vi "Write Best Cost.vi"(8 "error in (no error)":errorcluster, 10 "Best Cost":u64, 11 "State Value in":refnum<class "State Value.lvclass">) -> (0 "error out":errorcluster, 3 "State Value out":refnum<class "State Value.lvclass">)   [LabVIEW 2019, in "23.lvlib" / "State Value.lvclass"]
uses:
  State Value.lvclass
  State Value.lvclass/State Value.ctl
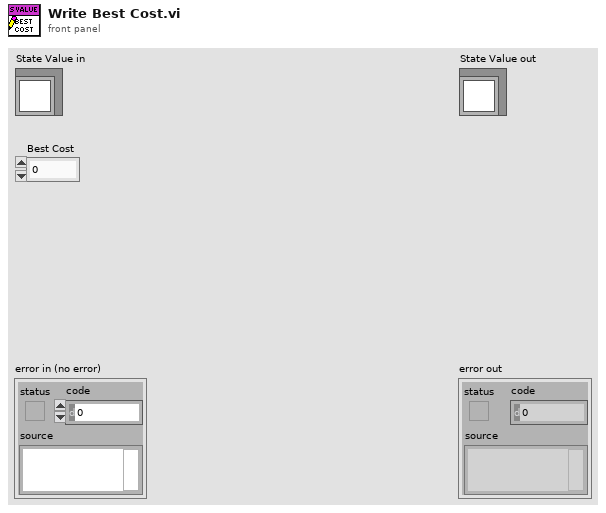
[diagram p1: front panel]
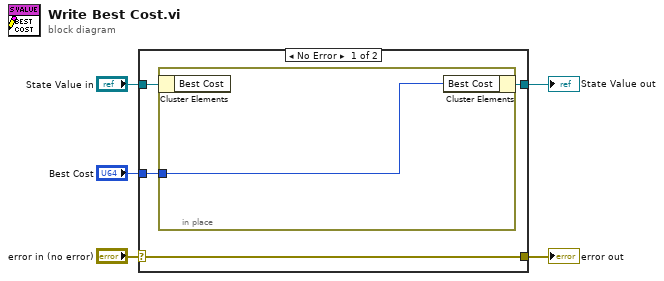
[diagram p0: block diagram]
diagram:
  n1 = case shown="No Error" "error in (no error)" {
    selector: "error in (no error)" -> [w9 w11]
    tunnel: [w9 w11] -> w4
    tunnel: [w7 w12] -> w2
    tunnel: "State Value in" -> [w6 w12]
    tunnel: "Best Cost" -> [w8 _]
    frame No Error {
      n2 = in-place {
        in-place-border: w8 -> [w10]
        n3 = in-place-cluster #1(w6) -> ()  [unwired: 1 out]
        n4 = in-place-cluster #1("Best Cost"=w10) -> (w7:refnum<class "State Value.lvclass">)
      }
    }
    frame Error {
    }
  }
  "error out" <- w4
  "State Value out" <- w2
